vi "Constants.vi"() -> ()   [LabVIEW 2017, in "Chassis TimeSync Shared.lvlib"]
doc: "Use this Global VI to access the GUIDs assigned to the page resources of the Custom Device."
uses:
  Chassis TimeSync Shared.lvlib
  Channel.ctl
panel:
  in  "Tab Control":enum32{"GUIDS", "Constants", "Properties"}(tab)=enum."Properties"
  in  "Chan Del Prot":string="C9C36D38-F811-822C-0C95-B5EFD5033E75"
  in  "Sect Del Prot":string="297B72C6-21C2-EA0B-6E7C-23F9EC8798A9"
  in  "Custom Device":string="85FE1586-82E1-A7AD-798B-5599EFFC50EE"
  in  "Mode:Custom":string="Specify entirely custom connections. Use the keyword \"Scan\" (without quotes) to specify scan sample clock as a source."
  in  "SysTime Section":string="System time"
  in  "Chassis Clock Section":string="Chassis Clock"
  in  "Master error":string="The Chassis TimeSync custom device at %s was configured to drive PXI_Trig0 but is not selected as the chassis master. Either change the drive connection or select this device as the chassis master."
  in  "Status Chans":T1[](array[typedef])=[{"Name"="Error code", "Units"="", "Default"=0.0, "Description"="Error code of the custom device. A negative value indicates failure. A positive value indicates warning."}]
  in  "TSModMissing Err":string="The Time-Based Synchronization Module name is missing."
  in  "TSModMissing":string="TSModMissing"
  in  "ChassisClk Chans":T1[](array[typedef])=[{"Name"="Synchronized", "Units"="", "Default"=0.0, "Description"=""}, {"Name"="Disruption Count", "Units"="", "Default"=0.0, "Description"=""}, {"Name"="Offset", "Units"="S", "Default"=0.0, "Description"="Offset in seconds of the pxi chassis clock time from the Time-Based synchronization module time"}]
  in  "Master type":string="Master type"
  in  "SysTime Chans":T1[](array[typedef])=[{"Name"="Synchronized", "Units"="", "Default"=0.0, "Description"=""}, {"Name"="Disruption Count", "Units"="", "Default"=0.0, "Description"=""}, {"Name"="Offset", "Units"="S", "Default"=0.0, "Description"="Offset in seconds of the system time from the Time-Based synchronization \n\nmodule time"}, {"Name"="Status", "Units"="", "Default"=0.0, "Description"="0: Good, 1: Unknown Error, 257: NI-Sync Device Not Found"}]
  in  "Mode:Route in":string="Routes an existing pulse on selected external pin to PXI_Trig0."
  in  "Mode:Route out":string="Routes an existing pulse on PXI_Trig0 to selected external pins."
  in  "Mode:Gen Sam":string="Generates a sample clock on selected pins. Pulses will be synchronous to EtherCAT (if present)."
  in  "PxiTrig1":string="PxiTrig1"
  in  "Clock and Trigger Routing":string="Clock and Trigger Routing"
  in  "CompiledData":string="CompiledData"
  in  "PPSStartTime":string="PPSStartTime"
  in  "PPSSetTime":string="PPSSetTime"
  in  "PPSTerminal":string="PPSTerminal"
  in  "IRIGType":string="IRIGType"
  in  "TimeRef":string="TimeRef"
  in  "Priority1":string="Priority1"
  in  "Priority2":string="Priority2"
  in  "SyncModule?":string="SyncModule?"
  in  "SyncModule":string="SyncModule"
  in  "RouteDest":string="RouteDest"
  in  "RouteSource":string="RouteSource"
  in  "ExternalPin":string="ExternalPin"
  in  "Pfi 2":string="Pfi 2"
  in  "Pfi 1":string="Pfi 1"
  in  "Pfi 0":string="Pfi 0"
  in  "PxiTrig":string="PxiTrig"
  in  "ConMode":string="ConMode"
  in  "ConSelection":string="ConSelection"
  in  "TimeKeeper":string="TimeKeeper"
  in  "StartDelay":string="StartDelay"
  in  "ScanOffset":string="ScanOffset"
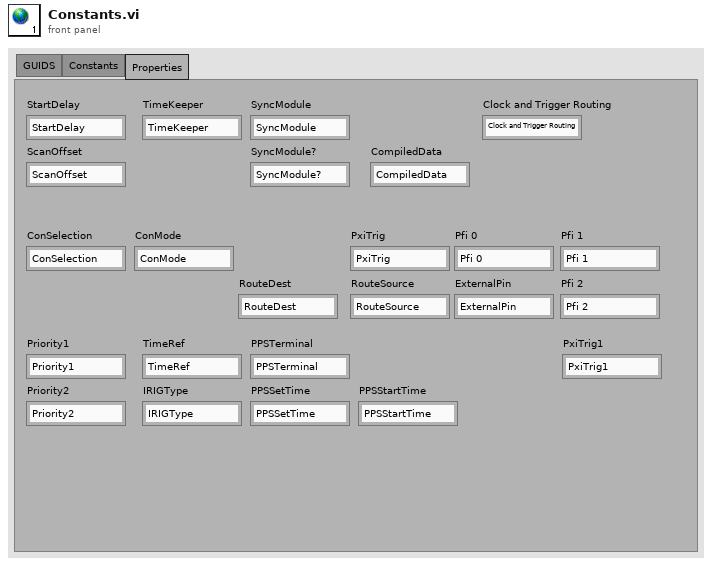
[diagram p1: front panel]
types:
  T1 = typedef "Chassis TimeSync Shared.lvlib/Channel.ctl" = cluster{"Name":string, "Units":string, "Default":dbl, "Description":string}
diagram:
